vi "PT (Main).vi"(7 "Name of Parent Panel":string="Main.vi", 9 "New Center Coords":T1={"Horizontal"=470, "Vertical"=200}, 10 "Config":variant, 11 "Main UI Message Queue":refnum<queue>) -> ()   [LabVIEW 2018, in "PT Module.lvlib"]
doc: "This Continuous Measurement sample project is based on the Queued Message Handler template.\n\nThe Event Handling Loop generates messages based on user interface actions.\n\nThe Message Handling Loop processes messages generated by the Event Handling Loop, or by other messages. There are also Acquisition and Logging message handling loop subVIs, and a chart updating loop."
uses:
  PT Module.lvlib
  support/Message Queue/Message Cluster.ctl
  <vilib>/Utility/miscctls.llb/LVPoint32TypeDef.ctl
  Controls/PT Module Config Cluster.ctl
  Tag VIs/Numeric Alarm Settings Cluster.ctl
  Tag VIs/Tag FGV Operation Enum.ctl
  support/Message Queue/Enqueue Message (Single).vi
  support/User Event - Stop/User Event - Stop.lvlib
  support/Support Library.lvlib
  support/Message Queue/Message Queue.lvlib
  Shared Variables/Dynamic Shared Variables.lvlib
  subVIs/PT Settings Dialog.vi
  support/Command Log VIs/Command Logging.lvlib
  Report Generation/Report Generation.lvlib
panel:
  in  "Settings":bool
  out "Display Cluster":cluster{"Tag Name":string, "Pressure":dbl} {"Pressure" format="%.1f"}
  out "H/W":dbl
  out "Original Height":u32
  out "Original Width":u32
  in  "Start":bool
  in  "Stop":bool
  out "Status":string
  in  "Exit":bool
  out "Input Channel Tag Name":string
  out "Log File path":path
  in  "Force Trigger":bool
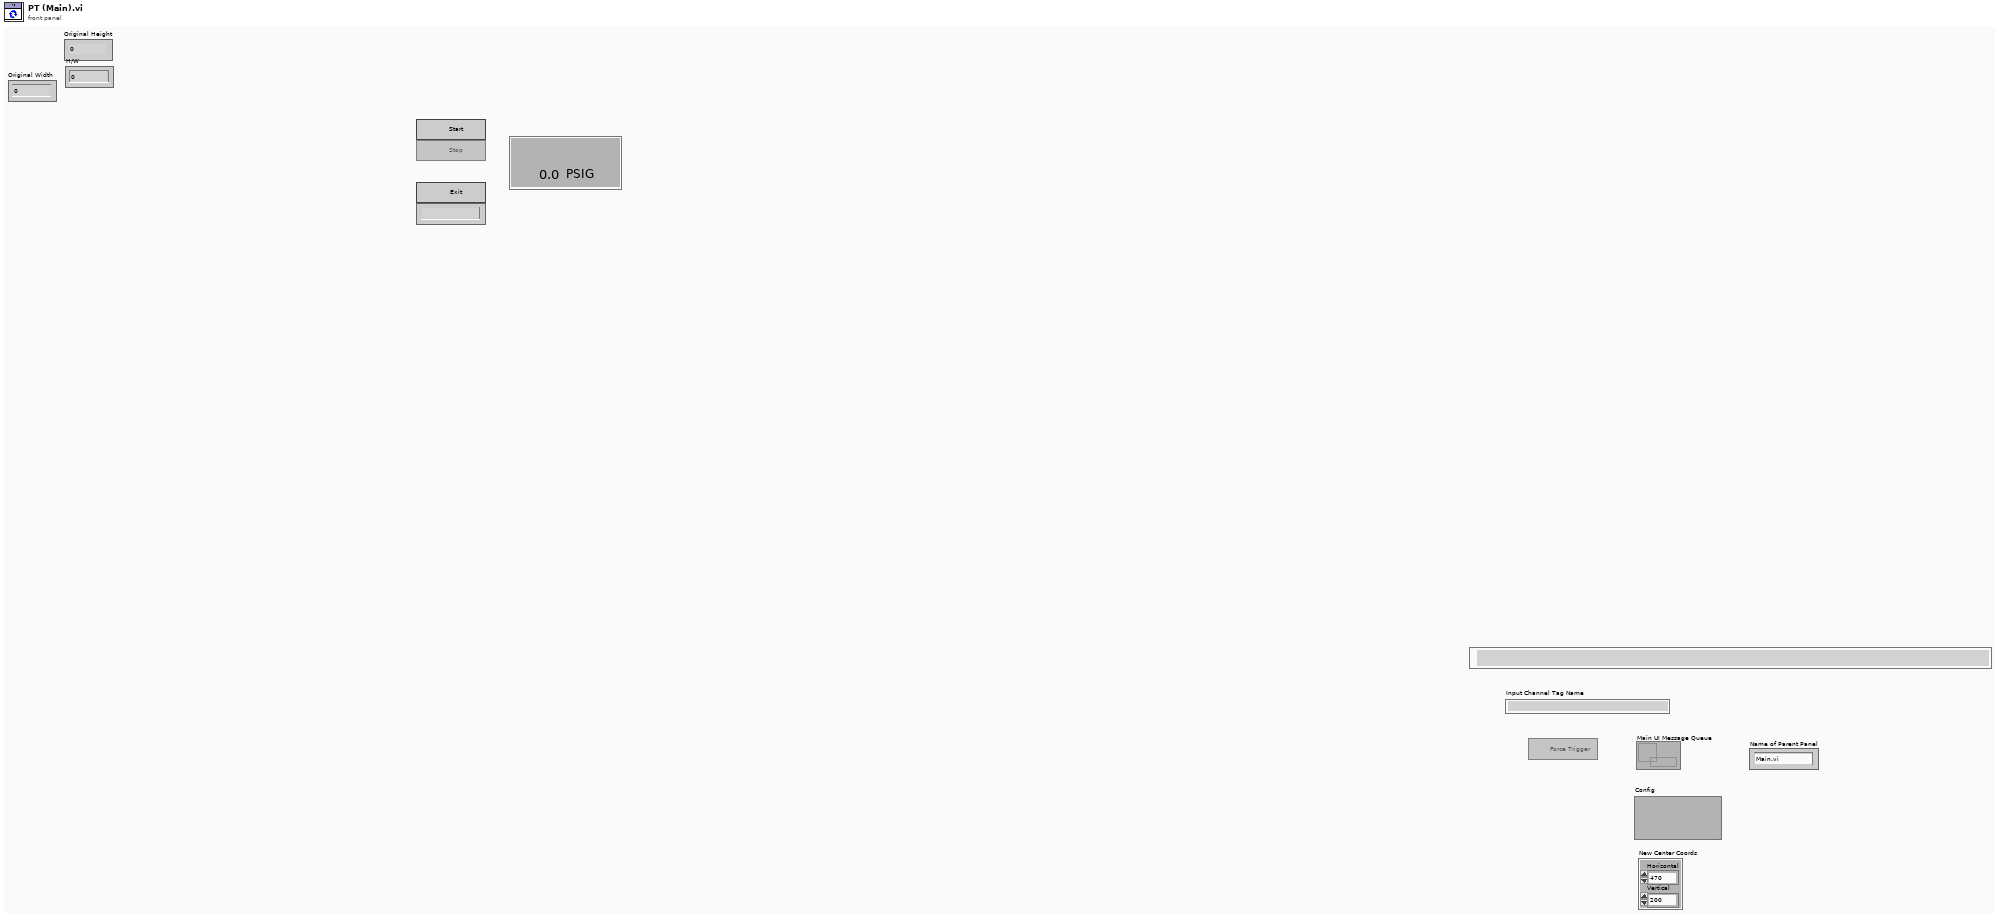
[diagram p1: front panel]
types:
  T1 = typedef "LVPoint32TypeDef.ctl" = cluster{"Horizontal":i32, "Vertical":i32}
  T2 = enum32{"Invalid", "Default", "Floating", "Floating/Auto-Hide", "Modal"}
  T3 = typedef "PT Module.lvlib/PT Module Config Cluster.ctl" = cluster{"GUID":string, "Drop Coords":T1, "Input Channel Tag Name ":string, "Process Name":string, "User name":string, "Queue Name":string, "Input Channel Numeric Alarm Settings":T4[]}
  T4 = typedef "Numeric Alarm Settings Cluster.ctl" = cluster{"enable? (F)":bool, "name":string, "alarm type":enum16{"HI_HI", "HI", "LO", "LO_LO"}, "level/change":dbl, "deadband/time":dbl, "alarm delay":dbl, "priority":u32, "ack type":enum16{"Auto", "User", "None", "Each Occurrence"}, "area":string, "description":string, "log? (T)":bool}
  T5 = typedef "LVPointTypeDef.ctl" = cluster{"Horizontal":i16, "Vertical":i16}
  T6 = typedef "Tag FGV Operation Enum.ctl" = enum16{"Init", "Set Notification Queue", "Create Tag", "Commit", "Write Tag (Numeric)", "Write Tag (Boolean)", "Read All Tags", "Read One Tag", "Delete Tag Category", "Set Alarm Parameters (Numeric)", "Set Alarm Parameters (Boolean)", "Enable All Alarms", "Disable All Alarms", "Delete All Tags", "Read Alarms", "Ack Alarm", "Read Alarm Parameters (Numeric)", "Read Alarm Parameters (Boolean)"}
  T7 = typedef "LVRectTypeDef.ctl" = cluster{"Left":i16, "Top":i16, "Right":i16, "Bottom":i16}
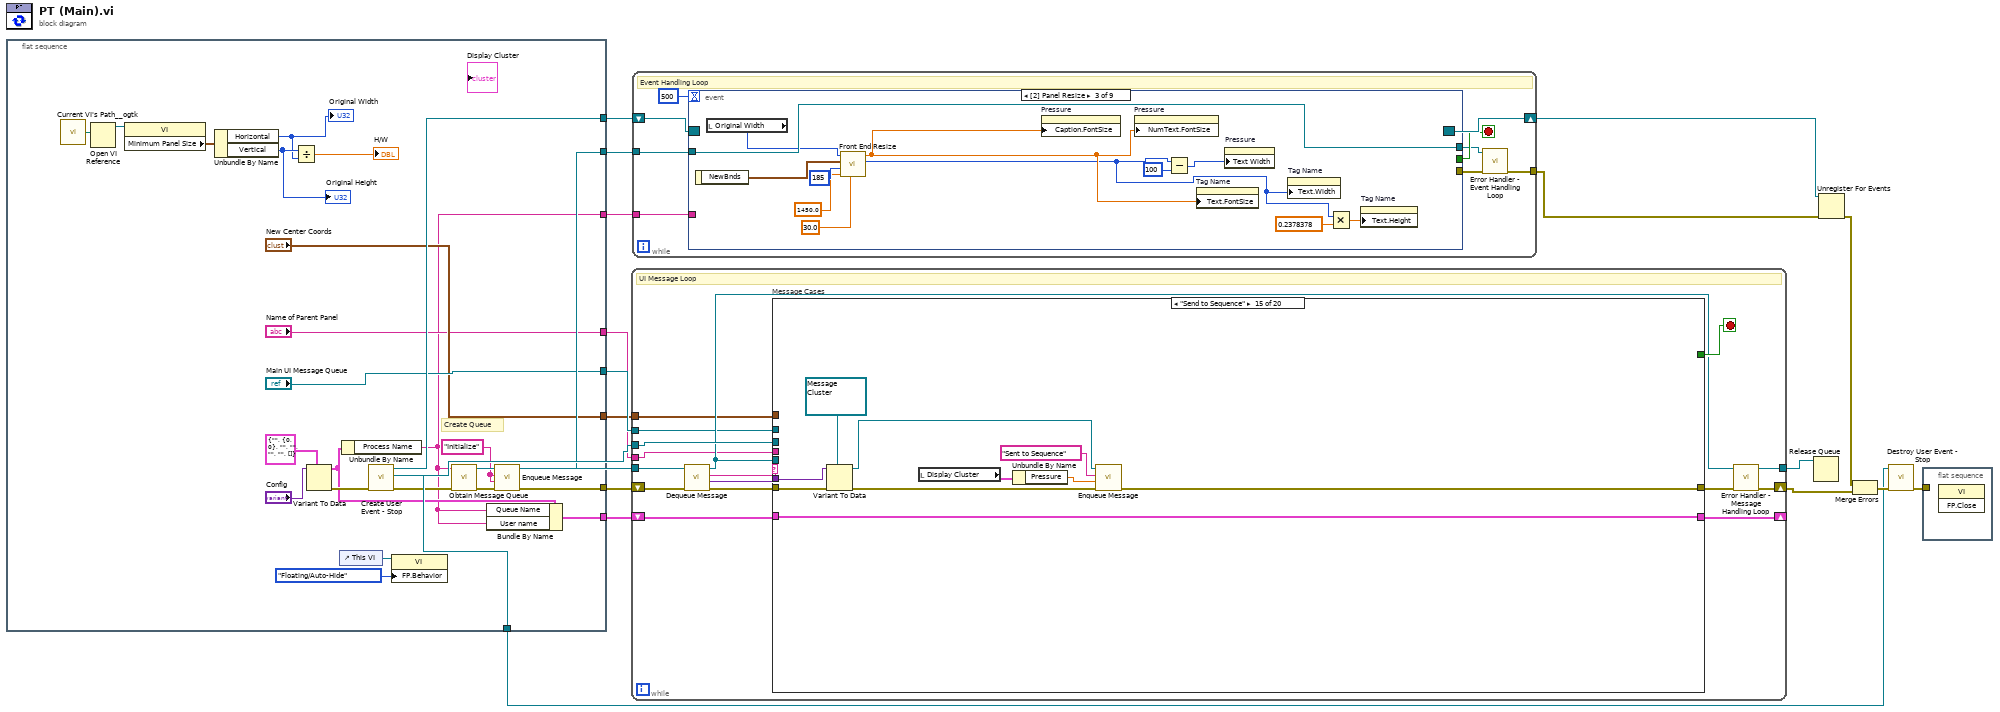
[diagram p0: block diagram]
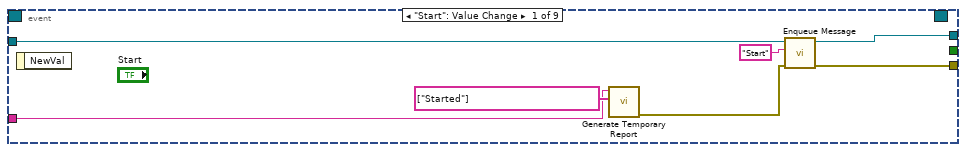
[diagram p2: hidden frame]
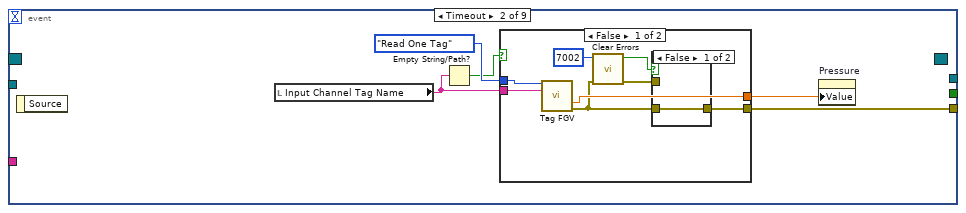
[diagram p3: hidden frame]
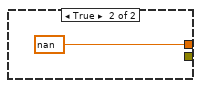
[diagram p5: hidden frame]
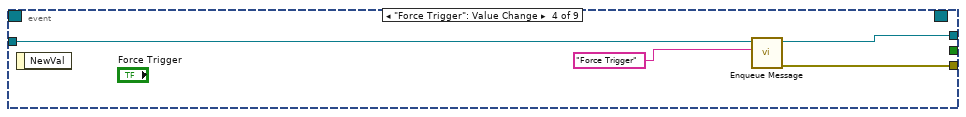
[diagram p6: hidden frame]
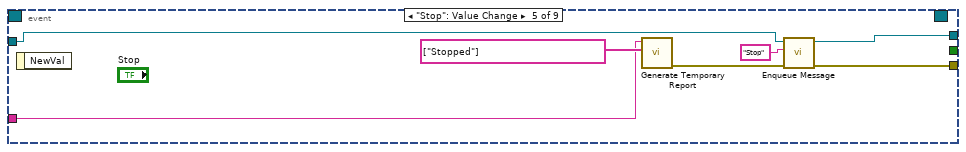
[diagram p7: hidden frame]
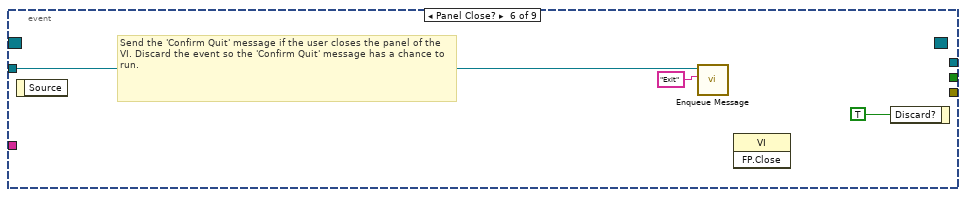
[diagram p8: hidden frame]
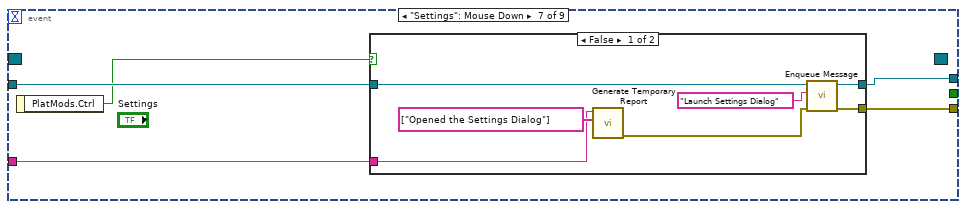
[diagram p9: hidden frame]
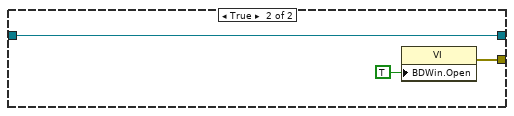
[diagram p10: hidden frame]
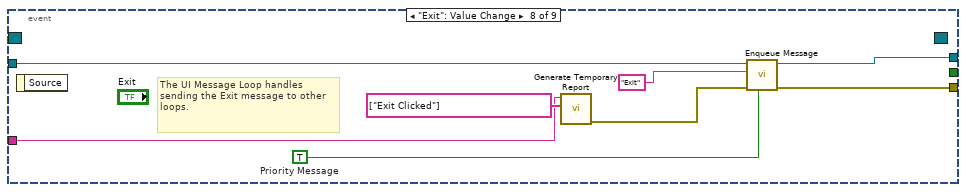
[diagram p11: hidden frame]
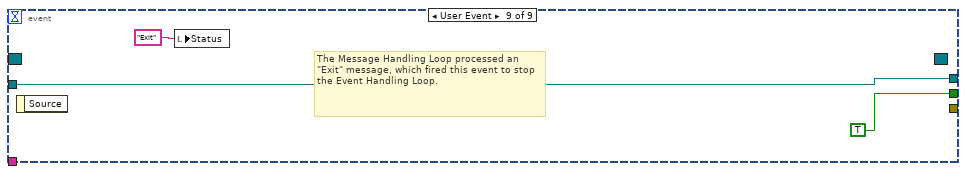
[diagram p12: hidden frame]
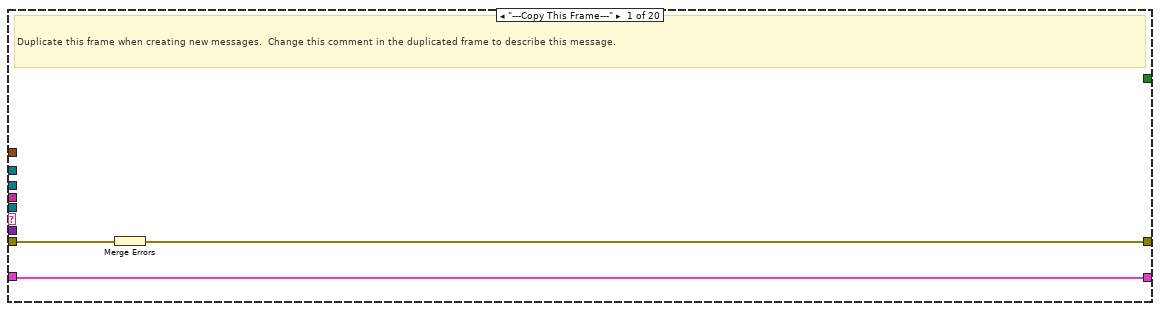
[diagram p13: hidden frame]
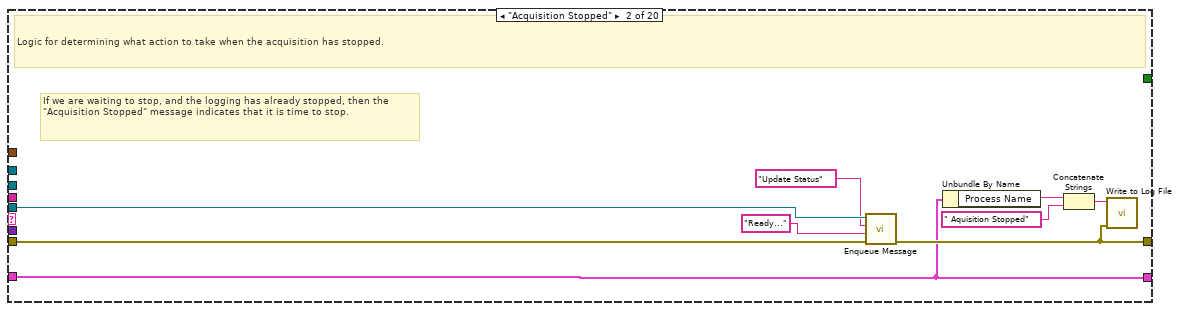
[diagram p14: hidden frame]
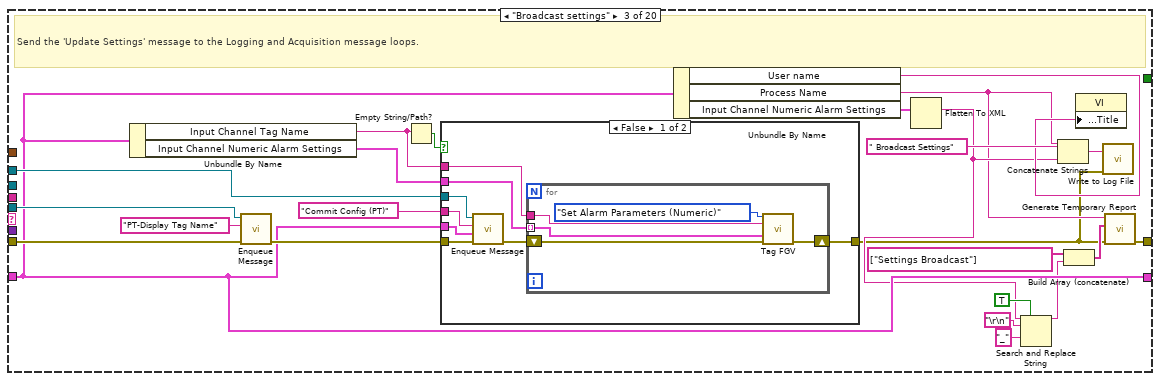
[diagram p15: hidden frame]
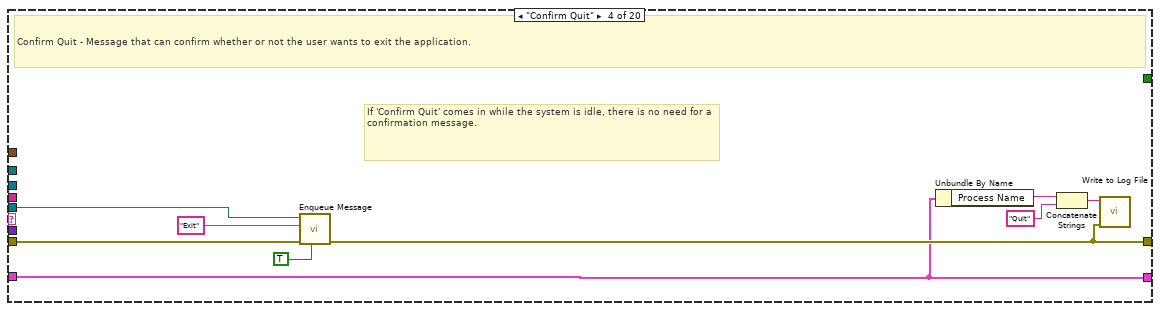
[diagram p17: hidden frame]
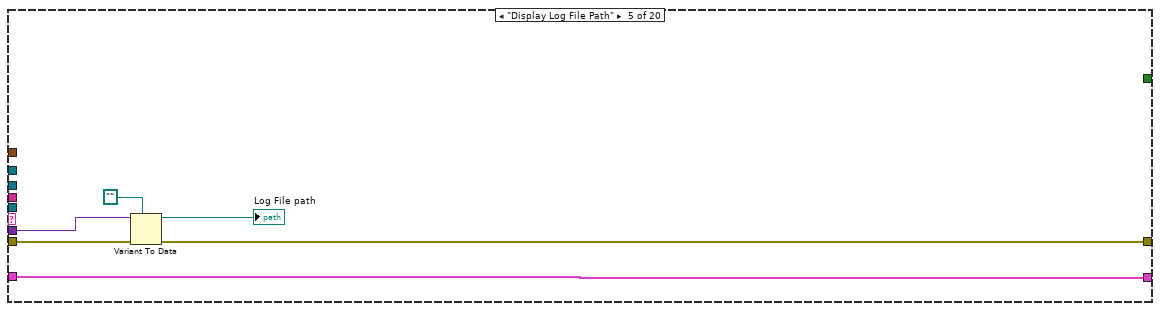
[diagram p18: hidden frame]
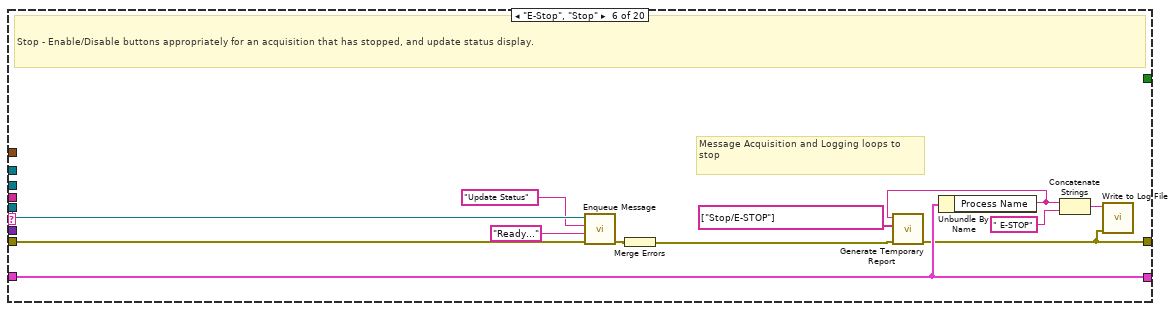
[diagram p19: hidden frame]
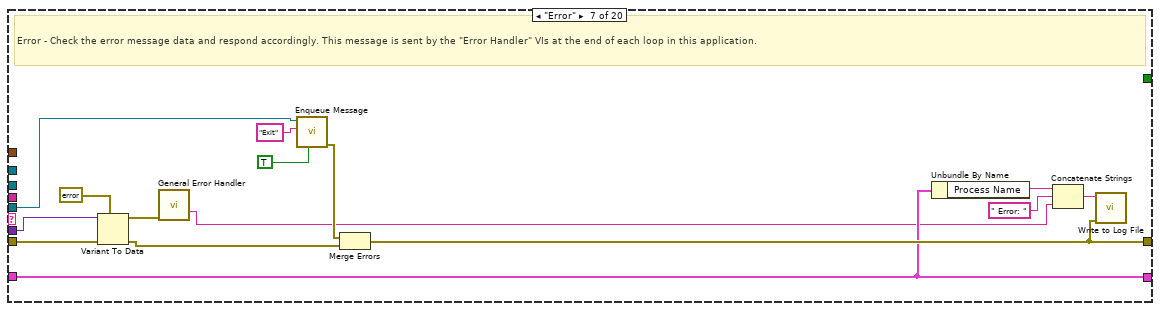
[diagram p20: hidden frame]
diagram:
  n1 = flat-sequence {
    tunnel: [w41] -> w14
    tunnel: [w40] -> w13
    tunnel: [w37] -> w10
    tunnel: [w35] -> w9
    tunnel: ["Main UI Message Queue"] -> w8
    tunnel: ["New Center Coords"] -> w7
    tunnel: ["Name of Parent Panel"] -> w6
    tunnel: [w26] -> w4
    tunnel: [w23] -> w1
    frame #0 {
      w36 = "Initialize" ("Message")
      # "Create Queue"
      n2 = call <userlib>:"Current VI's Path__ogtk.vi"() -> ("Current VI's Path (+ Relative)"=w18:path)  [unwired: 1 in]
      n3 = Open VI Reference(vi path=w18) -> (vi reference=w19:refnum<vi>)  [unwired: 5 in, 1 out]
      n4 = property class="VI"(reference=w19) -> ("Minimum Panel Size"=w20:T5)  [unwired: 1 in, 2 out]
      n5 = Unbundle By Name(w20) -> ("Horizontal"=w21:i16, "Vertical"=w22:i16)
      "Original Width" <- w21
      "Original Height" <- w22
      n6 = Divide(x=w22, y=w21) -> (x/y=→"H/W":dbl)
      n7 = Variant To Data(type=T3 {"GUID"="", "Drop Coords"={"Horizontal"=0, "Vertical"=0}, "Input Channel Tag Name "="", "Process Name"="", "User name"="", "Queue Name"="", "Input Channel Numeric Alarm Settings"=[]} ("TT Module Config"), Variant="Config") -> (data=w27:T3, error out=w30:errorcluster)  [unwired: 1 in]
      n8 = control-ref of="This VI"() -> (w25:refnum<vi>)
      n9 = Unbundle By Name(w27) -> ("Process Name"=w23:string)
      n10 = call "Create User Event - Stop.vi"("error in (no error)"=w30) -> ("error out"=w34:errorcluster, "User Event - Stop"=w40:refnum<user-event>, "Stop Event Registration Refnum"=w41:refnum<event-registration>)  [unwired: 8 in]
      n11 = property class="VI"(reference=w25, "FP.Behavior"=T2."Floating/Auto-Hide" ("Front Panel Window:Behavior")) -> ()  [unwired: 1 in, 2 out]
      n12 = call "Obtain Message Queue.vi"("error in (no error)"=w34, "name (unnamed)"=w23) -> ("error out"=w39:errorcluster, "Message Queue"=w38:refnum<queue>)  [unwired: 8 in]
      n13 = Bundle By Name(cluster=w27, "Queue Name"=w23, "User name"=w23) -> (w26:T3)
      n14 = call-poly "Enqueue Message.vi"("error in (no error)"=w39, "Message Data"=w36, "Message"=w36, "Message Queue"=w38) -> ("error out"=w35:errorcluster, "dup Message Queue"=w37:refnum<queue>)  [unwired: 6 in]
    }
  }
  n15 = while {
    tunnel: w10 -> [w51]
    tunnel: w13 -> [w56]
    shift-right: [w47] -> w3
    shift-left: w9 -> [w55]
    shift-right: [w50] -> _
    shift-left: w4 -> [w49]
    tunnel: w8 -> [w45]
    tunnel: w7 -> [w44]
    tunnel: w6 -> [w43]
    tunnel: [w42] -> w2
    stop <- w57 stop-if-true
    # "UI Message Loop"
    n16 = call "Dequeue Message.vi"("error in (no error)"=w55, "Message Queue"=w51) -> ("error out"=w54:errorcluster, "Message Data"=w52:variant, "Message"=w53:string, "dup Message Queue"=w46:refnum<queue>)  [unwired: 6 in]
    n17 = case "Message Cases" shown="\"Send to Sequence\"" w53 {
      selector: w53 -> [_ _ _ _ _ _ _ _ _ _ _ _ _ _ _ _ _ _ _ w271]
      tunnel: w46 -> [_ w68 w91 w116 _ w134 w145 w164 _ _ w203 w213 _ _ _ w245 _ _ _ _]
      tunnel: w54 -> [w60 w69 w93 w115 w117 w131 w149 w167 w173 w186 w200 w217 w223 w226 w231 w243 w253 w260 w268 _]
      tunnel: [w59 w62 w71 w109 w118 w124 w137 w150 w175 w186 w187 w209 w223 w226 w235 w239 w252 w259 w269 w270] -> w48
      tunnel: [_ _ _ _ _ _ _ TRUE _ _ _ _ _ _ _ _ _ _ _ _] -> w57
      tunnel: w52 -> [_ _ _ _ w120 _ w148 w157 _ _ _ _ _ _ w234 _ _ _ w267 _]
      tunnel: w56 -> [_ _ _ _ _ _ _ w166 _ _ _ _ _ _ _ _ _ _ _ _]
      tunnel: [w58 w61 w82 w108 w122 w127 w136 w154 w174 w185 w191 w208 w224 w227 w237 w240 w251 w255 w264 w276] -> w50
      tunnel: w49 -> [w58 w61 w82 w108 w122 w127 w136 w154 w174 w185 w191 w214 w224 w227 w237 w240 w251 w255 w264 w276]
      tunnel: w45 -> [_ _ w92 _ _ _ _ w158 _ _ _ _ _ _ _ _ _ w261 _ _]
      tunnel: w44 -> [_ _ _ _ _ _ _ _ _ _ w196 _ _ _ _ _ _ _ _ _]
      tunnel: w43 -> [_ _ _ _ _ _ _ _ _ _ w195 _ _ _ _ _ _ _ _ _]
      frame "---Copy This Frame---" {
        # "Duplicate this frame when creating new messages.  Change this comment in the duplicated frame to describe this message."
        n18 = Merge Errors(w60) -> (w59:errorcluster)
      }
      frame "Acquisition Stopped" {
        # "If we are waiting to stop, and the logging has already stopped, then the \"Acquisition Stopped\" message indicates that it is time to stop."
        # "Logic for determining what action to take when the acquisition has stopped."
        n19 = call-poly "Enqueue Message.vi"("error in (no error)"=w69, "Message Data"="Ready..." ("Message"), "Message"="Update Status", "Message Queue"=w68) -> ("error out"=w62:errorcluster)  [unwired: 6 in, 1 out]
        n20 = Unbundle By Name(w61) -> ("Process Name"=w65:string)
        n21 = Concatenate Strings(w65, " Aquisition Stopped" ("text")) -> (w64:string)
        n22 = call "Write to Log File.vi"("error in"=w62, "text"=w64) -> ()  [unwired: 9 in, 1 out]
      }
      frame "Broadcast settings" {
        # "Send the 'Update Settings' message to the Logging and Acquisition message loops."
        n23 = Unbundle By Name(w82) -> ("Input Channel Tag Name"=w85:string, "Input Channel Numeric Alarm Settings"=w89:T4[])
        n24 = call-poly "Enqueue Message.vi"("error in (no error)"=w93, "Message"="PT-Display Tag Name", "Message Queue"=w91) -> ("error out"=w87:errorcluster)  [unwired: 7 in, 1 out]
        n25 = Empty String/Path?(string/path=w85) -> (empty?=w88:bool)
        n26 = case shown="False" w88 {
          tunnel: w89 -> [w101 _]
          tunnel: [w100 w107] -> w70
          tunnel: w87 -> [w99 w107]
          tunnel: w82 -> [w98 _]
          tunnel: "Commit Config (PT)" ("Message") -> [w97 _]
          tunnel: w92 -> [w96 _]
          tunnel: w85 -> [w94 _]
          frame False {
            n27 = call-poly "Enqueue Message.vi"("error in (no error)"=w99, "Message Data"=w98, "Message"=w97, "Message Queue"=w96) -> ("error out"=w95:errorcluster)  [unwired: 6 in, 1 out]
            n28 = for {
              tunnel: w101 -> [w105] mode=indexing
              tunnel: w94 -> [w104]
              shift-right: [w102] -> w100
              shift-left: w95 -> [w103]
              n29 = call "Tag FGV.vi"("Operation"=Tag_FGV_Operation_Enum."Set Alarm Parameters (Numeric)", "Tag Name"=w104, "Data"=w105, "error in (no error)"=w103) -> ("error out"=w102:errorcluster)  [unwired: 4 in, 7 out]
            }
          }
          frame True {
          }
        }
        n30 = Unbundle By Name(w82) -> ("User name"=w80:string, "Process Name"=w72:string, "Input Channel Numeric Alarm Settings"=w81:T4[])
        n31 = Flatten To XML(anything=w81) -> (xml string=w75:string)
        n32 = Search and Replace String(replace all?=TRUE ("replace all? (F)"), input string=w75, search string="\r\n", replace string="_" ("replace string (\"\")")) -> (result string=w74:string)  [unwired: 4 in, 3 out]
        n33 = Concatenate Strings(w72, " Broadcast Settings" ("text"), w75) -> (w84:string)
        n34 = Build Array (concatenate)(string[] ["Settings Broadcast"] ("Line of Events"), w74) -> (w73:string[])
        n35 = property class="VI"("Front Panel.Title"=w80) -> ()  [unwired: 2 in, 2 out]
        n36 = call "Write to Log File.vi"("error in"=w70, "text"=w84) -> ()  [unwired: 9 in, 1 out]
        n37 = call "Generate Temporary Report.vi"("error in (no error)"=w70, "Line of Events"=w73, "Module Name"=w72) -> ("error out"=w71:errorcluster)  [unwired: 8 in]
      }
      frame "Confirm Quit" {
        # "If 'Confirm Quit' comes in while the system is idle, there is no need for a confirmation message."
        # "Confirm Quit - Message that can confirm whether or not the user wants to exit the application."
        n38 = call-poly "Enqueue Message.vi"("Priority Message? (F)"=TRUE, "error in (no error)"=w115, "Message"="Exit", "Message Queue"=w116) -> ("error out"=w109:errorcluster)  [unwired: 6 in, 1 out]
        n39 = Unbundle By Name(w108) -> ("Process Name"=w112:string)
        n40 = Concatenate Strings(w112, "Quit" ("text")) -> (w111:string)
        n41 = call "Write to Log File.vi"("error in"=w109, "text"=w111) -> ()  [unwired: 9 in, 1 out]
      }
      frame "Display Log File Path" {
        n42 = Variant To Data(error in=w117, type=path "", Variant=w120) -> (data=→"Log File path":path, error out=w118:errorcluster)
      }
      frame "E-Stop", "Stop" {
        # "Message Acquisition and Logging loops to stop"
        # "Stop - Enable/Disable buttons appropriately for an acquisition that has stopped, and update status display."
        n43 = call-poly "Enqueue Message.vi"("error in (no error)"=w131, "Message Data"="Ready..." ("Ready..."), "Message"="Update Status", "Message Queue"=w134) -> ("error out"=w130:errorcluster)  [unwired: 6 in, 1 out]
        n44 = Merge Errors(w130) -> (w125:errorcluster)
        n45 = Unbundle By Name(w127) -> ("Process Name"=w123:string)
        n46 = call "Generate Temporary Report.vi"("error in (no error)"=w125, "Line of Events"=string[] ["Stop/E-STOP"], "Module Name"=w123) -> ("error out"=w124:errorcluster)  [unwired: 8 in]
        n47 = Concatenate Strings(w123, " E-STOP" ("text")) -> (w129:string)
        n48 = call "Write to Log File.vi"("error in"=w124, "text"=w129) -> ()  [unwired: 9 in, 1 out]
      }
      frame "Error" {
        # "Error - Check the error message data and respond accordingly. This message is sent by the \"Error Handler\" VIs at the end of each loop in this application."
        n49 = Variant To Data(error in=w149, type=errorcluster {"status"=FALSE, "code"=0, "source"=""} ("error out"), Variant=w148) -> (data=w146:errorcluster, error out=w142:errorcluster)
        n50 = call <vilib>:"General Error Handler.vi"("error in (no error)"=w146) -> ("message"=w135:string)  [unwired: 10 in, 4 out]
        n51 = call-poly "Enqueue Message.vi"("Priority Message? (F)"=TRUE, "Message"="Exit", "Message Queue"=w145) -> ("error out"=w141:errorcluster)  [unwired: 7 in, 1 out]
        n52 = Merge Errors(w141, w142) -> (w137:errorcluster)
        n53 = Unbundle By Name(w136) -> ("Process Name"=w140:string)
        n54 = Concatenate Strings(w140, " Error: " ("text"), w135) -> (w139:string)
        n55 = call "Write to Log File.vi"("error in"=w137, "text"=w139) -> ()  [unwired: 9 in, 1 out]
      }
      frame "Exit" {
        w161 = TRUE  # Delete Module?
        # "Stop the VI"
        # "Exit - Fire the User Event to stop the Event Handling Loop.  Also send Exit messages to the Acquisition and Logging loops."
        n56 = Release Queue(queue=w164, error in (no error)=w167) -> (error out=w163:errorcluster)  [unwired: 1 in, 2 out]
        n57 = call "Fire User Event - Stop.vi"("User Event - Stop"=w166) -> ("error out"=w165:errorcluster)  [unwired: 10 in]
        n58 = Merge Errors(w165, w163) -> (w151:errorcluster)
        n59 = Variant To Data(type=w161, Variant=w157) -> (data=w160:bool, error out=w162:errorcluster)  [unwired: 1 in]
        n60 = Select(t=w161, s=w162, f=w160) -> (s? t:f=w159:bool)
        n61 = case "Don't enqueue Delete Module if opening campaign because it\nwill already have been deleted and new config loaded and we create\na race condition." shown="True" w159 {
          tunnel: w158 -> [_ w171]
          tunnel: w154 -> [_ w170]
          frame False {
          }
          frame True {
            n62 = Unbundle By Name(w170) -> ("GUID"=w169:string)
            n63 = call-poly "Enqueue Message.vi"("Message Data"=w169, "Message"="Delete Module", "Message Queue"=w171) -> ()  [unwired: 7 in, 2 out]
          }
        }
        n64 = Unbundle By Name(w154) -> ("Process Name"=w152:string)
        n65 = Concatenate Strings(w152, " Exit" ("text")) -> (w156:string)
        n66 = call "Generate Temporary Report.vi"("error in (no error)"=w151, "Line of Events"=string[] ["Exited"], "Module Name"=w152) -> ("error out"=w150:errorcluster)  [unwired: 8 in]
        n67 = call "Write to Log File.vi"("error in"=w150, "text"=w156) -> ()  [unwired: 9 in, 1 out]
      }
      frame "Force Trigger" {
        # "Force Trigger - send a message to the Logging message loop to start logging."
        n68 = Merge Errors(w173) -> (w175:errorcluster)
      }
      frame "Init UI Refs" {
        # "Init UI Refs - Store control references for UI controls.  Also enable/disable controls appropriately."
        n69 = control-ref of="Status"() -> ()  [unwired: 1 out]
        n70 = property class="VI"("Front Panel.Closeable"=TRUE ("Front Panel Window:Closeable")) -> ()  [unwired: 2 in, 2 out]
        n71 = control-ref of="Force Trigger"() -> (w178:refnum<vi>)
        n72 = control-ref of="Stop"() -> (w177:refnum<vi>)
        n73 = control-ref of="Exit"() -> (w179:refnum<vi>)
        n74 = control-ref of="Start"() -> (w182:refnum<vi>)
        n75 = Build Array(w177, w178) -> (w176:refnum<vi>[])
        n76 = Build Array(w179, w182) -> (w181:refnum<vi>[])
        n77 = call "Set Enable State on Multiple Controls.vi"("Enable?"=FALSE, "Controls"=w176) -> ()  [unwired: 10 in]
        n78 = call "Set Enable State on Multiple Controls.vi"("Enable?"=TRUE, "Controls"=w181) -> ()  [unwired: 10 in]
      }
      frame "Initialize" {
        # "Initialize - Get configuration settings, then message the UI to initialize, and broadcast the settings to the other message loops."
        n79 = Unbundle By Name(w191) -> ("Process Name"=w194:string)
        n80 = call-poly "Enqueue Message.vi"("error in (no error)"=w200, "Message"="Init UI Refs", "Message Queue"=w203) -> ("error out"=w201:errorcluster, "dup Message Queue"=w202:refnum<queue>)  [unwired: 7 in]
        n81 = property class="VI" props=["FP.State"]() -> (reference out=w197:refnum<vi>)  [unwired: 2 in, 2 out]
        n82 = call "Make Child and Move.vi"("Process Name"=w194, "Name of Parent Panel"=w195, "New Center Coords"=w196, "VI in"=w197) -> ()  [unwired: 8 in]
        n83 = call-poly "Enqueue Message.vi"("error in (no error)"=w201, "Message"="Broadcast Settings", "Message Queue"=w202) -> ("error out"=w198:errorcluster, "dup Message Queue"=w199:refnum<queue>)  [unwired: 7 in]
        n84 = call-poly "Enqueue Message.vi"("error in (no error)"=w198, "Message Data"="Ready..." ("Ready..."), "Message"="Update Status", "Message Queue"=w199) -> ("error out"=w188:errorcluster)  [unwired: 6 in, 1 out]
        n85 = Unbundle By Name(w191) -> ("Process Name"=w189:string)
        n86 = call "Generate Temporary Report.vi"("error in (no error)"=w188, "Line of Events"=string[] ["Initialized"], "Module Name"=w189) -> ("error out"=w187:errorcluster)  [unwired: 8 in]
        n87 = Concatenate Strings(w189, " Initialize" ("text")) -> (w193:string)
        n88 = call "Write to Log File.vi"("error in"=w187, "text"=w193) -> ()  [unwired: 9 in, 1 out]
      }
      frame "Launch Settings Dialog" {
        # "Launch the Settings Dialog when the user clicks the 'Settings' button."
        n89 = call-by-ref "?"("error in (no error)"=w217, "PT Module Config in"=w214) -> ("error out"=w215:errorcluster, "Cancelled?"=w216:bool, "PT Module Config out"=w208:T3)  [unwired: 8 in, 3 out]
        n90 = case shown="False" w216 {
          tunnel: w215 -> [w219 w222]
          tunnel: [w221 w222] -> w209
          tunnel: w208 -> [_ _]
          tunnel: w213 -> [w218 _]
          frame False {
            n91 = call-poly "Enqueue Message.vi"("error in (no error)"=w219, "Message"="Broadcast settings", "Message Queue"=w218) -> ("error out"=w221:errorcluster)  [unwired: 7 in, 1 out]
          }
          frame True {
          }
        }
        n92 = Unbundle By Name(w208) -> ("Process Name"=w212:string)
        n93 = Concatenate Strings(w212, " Settings Dialog Launched" ("text")) -> (w211:string)
        n94 = call "Write to Log File.vi"("error in"=w209, "text"=w211) -> ()  [unwired: 9 in, 1 out]
      }
      frame "Logging Stopped" {
        # "Logic for determining what action to take when the logging has stopped."
      }
      frame "PT-Display Tag Name" {
        n95 = Unbundle By Name(w227) -> ("Input Channel Tag Name"=w225:string)
        "Input Channel Tag Name" <- w225
        n96 = property on="Tag Name" class="Str"("Text.Text"=w225) -> ()  [unwired: 2 in, 2 out]
      }
      frame "Send to Sequence" {
        n97 = Variant To Data(error in=w231, type=refnum<queue> refnum ("Message Queue"), Variant=w234) -> (data=w232:refnum<queue>, error out=w230:errorcluster)
        n98 = local read "Display Cluster"() -> (w229:cluster{"Tag Name":string, "Pressure":dbl})
        n99 = Unbundle By Name(w229) -> ("Pressure"=w228:dbl)
        n100 = call-poly "Enqueue Message.vi"("error in (no error)"=w230, "Message Data"=w228, "Message"="Sent to Sequence", "Message Queue"=w232) -> ("error out"=w235:errorcluster)  [unwired: 6 in, 1 out]
      }
      frame "Start" {
        # "Message Acquisition and Logging loops to start"
        # "Start - Enable/Disable buttons appropriately for an acquisition that has started, and update status display."
        n101 = call-poly "Enqueue Message.vi"("error in (no error)"=w243, "Message"="Broadcast settings", "Message Queue"=w245) -> ("error out"=w246:errorcluster, "dup Message Queue"=w244:refnum<queue>)  [unwired: 7 in]
        n102 = call-poly "Enqueue Message.vi"("error in (no error)"=w246, "Message"="Start Loops", "Message Queue"=w244) -> ("error out"=w247:errorcluster)  [unwired: 7 in, 1 out]
        n103 = Merge Errors(w247) -> (w239:errorcluster)
        n104 = Unbundle By Name(w240) -> ("Process Name"=w238:string)
        n105 = Concatenate Strings(w238, " Start" ("text")) -> (w242:string)
        n106 = call "Write to Log File.vi"("error in"=w239, "text"=w242) -> ()  [unwired: 9 in, 1 out]
      }
      frame "Start Loops" {
        # "Message Acquisition and Logging loops to start"
        # "Start - Enable/Disable buttons appropriately for an acquisition that has started, and update status display."
        n107 = Unbundle By Name(w251) -> ("Process Name"=w250:string)
        n108 = call "Generate Temporary Report.vi"("error in (no error)"=w253, "Line of Events"=string[] ["Started"], "Module Name"=w250) -> ("error out"=w252:errorcluster)  [unwired: 8 in]
      }
      frame "Start Log" {
        # "The Tags are created in the DAQ Loop, but we need the \"Tags Created\" message count to = the # of modules dropped."
        n109 = call-poly "Enqueue Message.vi"("error in (no error)"=w260, "Message"="Tags Created", "Message Queue"=w261) -> ("error out"=w259:errorcluster)  [unwired: 7 in, 1 out]
        n110 = Unbundle By Name(w255) -> ("Process Name"=w258:string)
        n111 = Concatenate Strings(w258, " Tags Made" ("text")) -> (w257:string)
        n112 = call "Write to Log File.vi"("text"=w257) -> ()  [unwired: 10 in, 1 out]
      }
      frame "Update Status" {
        # "Update Display - Convert the message data to a string to display in the Status indicator."
        n113 = Variant To Data(error in=w268, type="", Variant=w267) -> (data=→"Status":string, error out=w265:errorcluster)
        n114 = Merge Errors(w265) -> (w269:errorcluster)
      }
      frame Default {
        # "'Default' case only runs if there is a message that isn't defined in any of the other cases.  Output a programming error."
        n115 = Concatenate Strings("The invalid message string " ("string"), w271, " was received in PT Main." ("string")) -> (w272:string)
        n116 = Bundle By Name(cluster=errorcluster {"status"=TRUE, "code"=1, "source"=""} ("error constant"), "source"=w272) -> (w270:errorcluster)
        n117 = Unbundle By Name(w276) -> ("Process Name"=w279:string)
        n118 = Concatenate Strings(w279, " Incorrect Message Received" ("text"), w271) -> (w278:string)
        n119 = call "Write to Log File.vi"("error in"=w270, "text"=w278) -> ()  [unwired: 9 in, 1 out]
      }
    }
    n120 = call "Error Handler - Message Handling Loop.vi"("error in (no error)"=w48, "Message Queue"=w46) -> ("dup error in"=w47:errorcluster, "dup Message Queue"=w42:refnum<queue>)  [unwired: 8 in]
  }
  n121 = while {
    tunnel: w10 -> [w287]
    tunnel: [w282] -> w16
    shift-right: [w286] -> w11
    shift-left: w14 -> [w288]
    tunnel: w1 -> [w280]
    stop <- w285 stop-if-true
    # "Event Handling Loop"
    n122 = event shown="[2] Panel Resize" {
      selector: w288 -> [_ _ _ _ _ _ _ _ _]
      dyn-events: [_ _ _ _ _ _ _ _ _] -> w286
      timeout: 500 -> [_ _ _ _ _ _ _ _ _]
      tunnel: [_ _ _ _ _ _ _ _ TRUE ("Discard?")] -> w285
      tunnel: w287 -> [w293 _ w319 w326 w333 w335 w341 w357 w361]
      tunnel: [w295 w299 _ w325 w332 _ w342 w360 _] -> w283
      tunnel: [w292 _ w319 w324 w331 _ w340 w356 w361] -> w284
      tunnel: w280 -> [w290 _ _ _ w329 _ w338 w354 _]
      event "Start": Value Change {
        n123 = event-data() -> ()  [unwired: 1 in, 1 out]
        n124 = call "Generate Temporary Report.vi"("Line of Events"=string[] ["Started"], "Module Name"=w290) -> ("error out"=w289:errorcluster)  [unwired: 9 in]
        n125 = call-poly "Enqueue Message.vi"("error in (no error)"=w289, "Message"="Start", "Message Queue"=w293) -> ("error out"=w295:errorcluster, "dup Message Queue"=w292:refnum<queue>)  [unwired: 7 in]
      }
      event Timeout {
        n126 = event-data() -> ()  [unwired: 1 in, 1 out]
        n127 = local read "Input Channel Tag Name"() -> (w298:string)
        n128 = Empty String/Path?(string/path=w298) -> (empty?=w297:bool)
        n129 = case shown="False" w297 {
          tunnel: Tag_FGV_Operation_Enum."Read One Tag" ("Operation") -> [w308 _]
          tunnel: [w307 nan ("Tag Value")] -> w296
          tunnel: [w302 _] -> w299
          tunnel: w298 -> [w306 _]
          frame False {
            n130 = call "Tag FGV.vi"("Operation"=w308, "Tag Name"=w306) -> ("Tag Value"=w307:dbl, "error out"=w301:errorcluster)  [unwired: 6 in, 6 out]
            n131 = call <vilib>:"Clear Errors.vi"("error in (no error)"=w301, "specific error code to clear (0: all)"=7002) -> ("error out"=w303:errorcluster, "specific error cleared?"=w304:bool)  [unwired: 4 in]
            n132 = case shown="False" w304 {
              tunnel: [w309 w310] -> w302
              tunnel: w303 -> [_ w310]
              tunnel: w301 -> [w309 _]
              frame False {
              }
              frame True {
              }
            }
          }
          frame True {
          }
        }
        n133 = property on="Pressure" class="DigNum (strict)"("Value"=w296) -> ()  [unwired: 2 in, 2 out]
      }
      event Panel Resize {
        n134 = event-data() -> ("NewBnds"=w320:T7)  [unwired: 1 in]
        n135 = local read "Original Width"() -> (w318:u32)
        n136 = call "Front End Resize.vi"("Starting Font"=30.0, "Area to Font Division"=1450.0, "Original Text Box Width"=185, "NewBnds"=w320, "Original Panel Width"=w318) -> ("New Text Box Width"=w312:u64, "New Font Size"=w313:dbl)  [unwired: 5 in]
        n137 = property on="Pressure" class="DigNum (strict)"("Caption.FontSize"=w313) -> ()  [unwired: 2 in, 2 out]
        n138 = property on="Pressure" class="DigNum (strict)"("NumText.FontSize"=w313) -> ()  [unwired: 2 in, 2 out]
        n139 = Subtract(x=w312, y=u64 100) -> (x-y=w316:u64)
        n140 = property on="Tag Name" class="Str"("Text.FontSize"=w313) -> ()  [unwired: 2 in, 2 out]
        n141 = property on="Pressure" class="DigNum (strict)"("Text Width"=w316) -> ()  [unwired: 2 in, 2 out]
        n142 = property on="Tag Name" class="Str"("Text.Width"=w312) -> ()  [unwired: 2 in, 2 out]
        n143 = Multiply(x=w312, y=0.2378378 ("Starting Font")) -> (x*y=w315:dbl)
        n144 = property on="Tag Name" class="Str"("Text.Height"=w315) -> ()  [unwired: 2 in, 2 out]
      }
      event "Force Trigger": Value Change {
        n145 = event-data() -> ()  [unwired: 1 in, 1 out]
        n146 = call-poly "Enqueue Message.vi"("Message"="Force Trigger", "Message Queue"=w326) -> ("error out"=w325:errorcluster, "dup Message Queue"=w324:refnum<queue>)  [unwired: 8 in]
      }
      event "Stop": Value Change {
        n147 = event-data() -> ()  [unwired: 1 in, 1 out]
        n148 = call "Generate Temporary Report.vi"("Line of Events"=string[] ["Stopped"], "Module Name"=w329) -> ("error out"=w328:errorcluster)  [unwired: 9 in]
        n149 = call-poly "Enqueue Message.vi"("error in (no error)"=w328, "Message"="Stop", "Message Queue"=w333) -> ("error out"=w332:errorcluster, "dup Message Queue"=w331:refnum<queue>)  [unwired: 7 in]
      }
      event Panel Close? {
        # "Send the 'Confirm Quit' message if the user closes the panel of the VI. Discard the event so the 'Confirm Quit' message has a chance to run."
        n150 = event-data() -> ()  [unwired: 1 in, 1 out]
        n151 = call-poly "Enqueue Message.vi"("Message"="Exit", "Message Queue"=w335) -> ()  [unwired: 8 in, 2 out]
        n152 = invoke class="VI" method="FP.Close"() -> ()  [unwired: 3 in, 3 out]
        n153 = event-data("Discard?"=TRUE) -> ()  [unwired: 1 in, 1 out]
      }
      event "Settings": Mouse Down {
        n154 = event-data() -> ("PlatMods.Ctrl"=w339:bool)  [unwired: 1 in]
        n155 = case shown="False" w339 {
          tunnel: [w349 w351] -> w342
          tunnel: w341 -> [w347 w350]
          tunnel: [w346 w350] -> w340
          tunnel: w338 -> [w344 _]
          frame False {
            n156 = call "Generate Temporary Report.vi"("Line of Events"=string[] ["Opened the Settings Dialog"], "Module Name"=w344) -> ("error out"=w343:errorcluster)  [unwired: 9 in]
            n157 = call-poly "Enqueue Message.vi"("error in (no error)"=w343, "Message"="Launch Settings Dialog", "Message Queue"=w347) -> ("error out"=w349:errorcluster, "dup Message Queue"=w346:refnum<queue>)  [unwired: 7 in]
          }
          frame True {
            n158 = property class="VI"("BDWin.Open"=TRUE ("Block Diagram Window:Open")) -> (error out=w351:errorcluster)  [unwired: 2 in, 1 out]
          }
        }
      }
      event "Exit": Value Change {
        w358 = TRUE  # Priority Message
        # "The UI Message Loop handles sending the Exit message to other loops."
        n159 = event-data() -> ()  [unwired: 1 in, 1 out]
        n160 = call "Generate Temporary Report.vi"("Line of Events"=string[] ["Exit Clicked"], "Module Name"=w354) -> ("error out"=w353:errorcluster)  [unwired: 9 in]
        n161 = call-poly "Enqueue Message.vi"("Priority Message? (F)"=w358, "error in (no error)"=w353, "Message"="Exit", "Message Queue"=w357) -> ("error out"=w360:errorcluster, "dup Message Queue"=w356:refnum<queue>)  [unwired: 6 in]
      }
      event User Event {
        # "The Message Handling Loop processed an \"Exit\" message, which fired this event to stop the Event Handling Loop."
        n162 = event-data() -> ()  [unwired: 1 in, 1 out]
        n163 = local write "Status"("Exit" ("Exit String")) -> ()
      }
    }
    n164 = call "Error Handler - Event Handling Loop.vi"("error in (no error)"=w283, "Message Queue"=w284) -> ("dup error in"=w282:errorcluster)  [unwired: 8 in, 1 out]
  }
  n165 = Release Queue(queue=w2) -> ()  [unwired: 2 in, 3 out]
  n166 = Unregister For Events(event registration refnum=w11, error in=w16) -> (error out=w12:errorcluster)
  n167 = Merge Errors(w12, w3) -> (w15:errorcluster)
  n168 = call "Destroy User Event - Stop.vi"("error in (no error)"=w15, "User Event - Stop"=w13) -> ("error out"=w5:errorcluster)  [unwired: 9 in]
  n169 = flat-sequence {
    tunnel: w5 -> [_]
    frame #0 {
      n170 = invoke class="VI" method="FP.Close"() -> ()  [unwired: 3 in, 3 out]
    }
  }
